vi "LoadDataHelper.vi"() -> (0 "Time Resolution [ms/pixel]":dbl format="%.2f", 1 "pixel per line":u32, 2 "planes":u32, 3 "lines":u32, 4 "Retrace":bool)   [LabVIEW 2009]
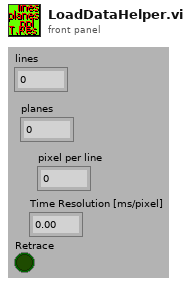
[diagram p1: front panel]
types:
  T1 = typedef "ImageSettings.ctt" = cluster{"Start Position (µm)":cluster{"x":dbl, "y":dbl, "z":dbl}, "End Position (µm)":cluster{"x":dbl, "y":dbl, "z":dbl}, "Image Resolution (nm/pixel)":cluster{"x":dbl, "y":dbl, "z":dbl}, "Image Size (µm)":cluster{"x":dbl, "y":dbl, "z":dbl}, "Image Size (pixel)":cluster{"x":u32, "y":u32, "z":u32}, "Time Resolution\n(ms/pixel)":dbl, "1st Axis":u16, "2nd Axis":u16, "Retrace":bool, "Estimated Time":string}
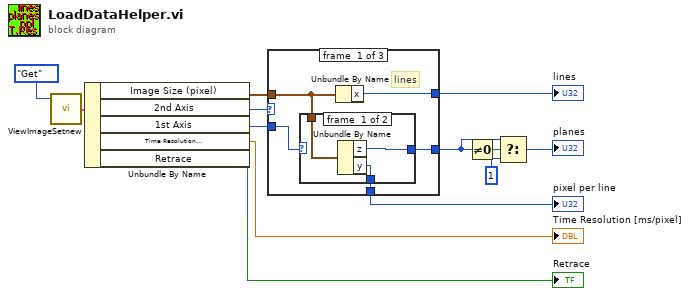
[diagram p0: block diagram]
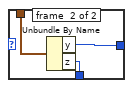
[diagram p2: hidden frame]
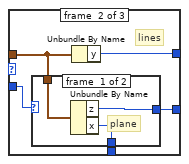
[diagram p3: hidden frame]
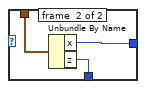
[diagram p4: hidden frame]
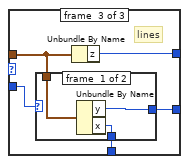
[diagram p5: hidden frame]
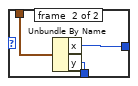
[diagram p6: hidden frame]
diagram:
  n1 = call "ViewImageSetnew.vi"("action"=enum16{"Display", "change", "Get", "Set"}."Get" ("Enum")) -> ("Image Settings"=w9:T1)  [unwired: 2 in]
  n2 = Unbundle By Name(w9) -> ("Image Size (pixel)"=w6:cluster{"x":u32, "y":u32, "z":u32}, "2nd Axis"=w7:u16, "1st Axis"=w8:u16, "Time Resolution\n(ms/pixel)"=→"Time Resolution [ms/pixel]":dbl, "Retrace"=→"Retrace":bool)
  n3 = case shown="1" w7 {
    tunnel: w6 -> [w16 w28 w38]
    tunnel: [w18 w29 w40] -> w13
    tunnel: w8 -> [w17 w26 w39]
    tunnel: [w15 w27 w37] -> w2
    tunnel: [w14 w25 w36] -> w11
    frame #0 {
      # "lines"
      n4 = case shown="1, Default" w17 {
        tunnel: w16 -> [w21 w24]
        tunnel: [w20 w23] -> w15
        tunnel: [w19 w22] -> w14
        frame #0 {
          n5 = Unbundle By Name(w21) -> ("z"=w20:u32, "y"=w19:u32)
        }
        frame #1 {
          n6 = Unbundle By Name(w24) -> ("y"=w23:u32, "z"=w22:u32)
        }
      }
      n7 = Unbundle By Name(w16) -> ("x"=w18:u32)
    }
    frame #1 {
      # "lines"
      n8 = case shown="0, Default" w26 {
        tunnel: w28 -> [w32 w35]
        tunnel: [w31 w34] -> w27
        tunnel: [w30 w33] -> w25
        frame #0 {
          # "plane"
          n9 = Unbundle By Name(w32) -> ("z"=w31:u32, "x"=w30:u32)
        }
        frame #1 {
          n10 = Unbundle By Name(w35) -> ("x"=w34:u32, "z"=w33:u32)
        }
      }
      n11 = Unbundle By Name(w28) -> ("y"=w29:u32)
    }
    frame #2 {
      # "lines"
      n12 = case shown="0, Default" w39 {
        tunnel: w38 -> [w43 w46]
        tunnel: [w42 w45] -> w37
        tunnel: [w41 w44] -> w36
        frame #0 {
          n13 = Unbundle By Name(w43) -> ("y"=w42:u32, "x"=w41:u32)
        }
        frame #1 {
          n14 = Unbundle By Name(w46) -> ("x"=w45:u32, "y"=w44:u32)
        }
      }
      n15 = Unbundle By Name(w38) -> ("z"=w40:u32)
    }
  }
  "lines" <- w13
  "pixel per line" <- w11
  n16 = Not Equal To 0?(x=w2) -> (x != 0?=w3:bool)
  n17 = Select(t=w2, s=w3, f=u32 1) -> (s? t:f=→"planes":u32)
